vi "Test Query Auth.vi"() -> ()   [LabVIEW 2020]
uses:
  HTTP Server/Trace Log.ctl
  HTTP Server/Trace Item.ctl
  HTTP Server/Processing Step.ctl
  <vilib>/IlluminatedG/IG HTTP Utils/HTTP Utils/Method.ctl
  TestQueryAuth/TestQueryAuth.lvclass
  C:/dev/IlluminatedG/lv-http-server/HTTP Server/Handler/Handler.lvclass
  QueryAuthController/QueryAuthController.lvclass
  HTTP Server/Server/Add Connection Handler.vi
  HTTP Server/Server/Add Request Handler.vi
  HTTP Server/Server/Add Route Handler.vi
  HTTP Server/Server/Add Controller Handler.vi
  HTTP Server/Server/Add Controller.vi
  HTTP Server/Server/Add Response Handler.vi
  HTTP Server/Server/Add Complete Handler.vi
  HTTP Server/Server/Add Exception Handler.vi
  HTTP Server/Connection Handler/Connection Handler.lvclass
  HTTP Server/Request Handler/Request Handler.lvclass
  HTTP Server/Route Handler/Route Handler.lvclass
  HTTP Server/Controller Handler/Controller Handler.lvclass
  HTTP Server/Controller/Controller.lvclass
  HTTP Server/Response Handler/Response Handler.lvclass
  HTTP Server/Complete Handler/Complete Handler.lvclass
  HTTP Server/Exception Handler/Exception Handler.lvclass
  HTTP Server/Server/Server.lvclass
  HTTP Server/Handler/Handler.lvclass
  HTTP Server/RequestTraceLog/RequestTraceLog.lvclass
  HTTP Server/HTTP Server.lvlib
  <vilib>/IlluminatedG/IG HTTP Utils/HTTP Utils/HTTP Utils.lvlib
panel:
  in  "Refresh Traces":bool
  out "Traces":T1[](array[typedef]) {"Sending" format="%_6f"; "Expires" format="%<%X %x>T"; "Created" format="%<%X %x>T"; "Waiting" format="%_6f"; "Parsing" format="%_6f"; "Processing" format="%_6f"; "Items"."Time" format="%.6f"; "Items"."Duration" format="%.6f"}
  out "error out":errorcluster
  in  "Port":u16=36987
  # "Request"
  # "Response"
  # "Session"
  # "Auth"
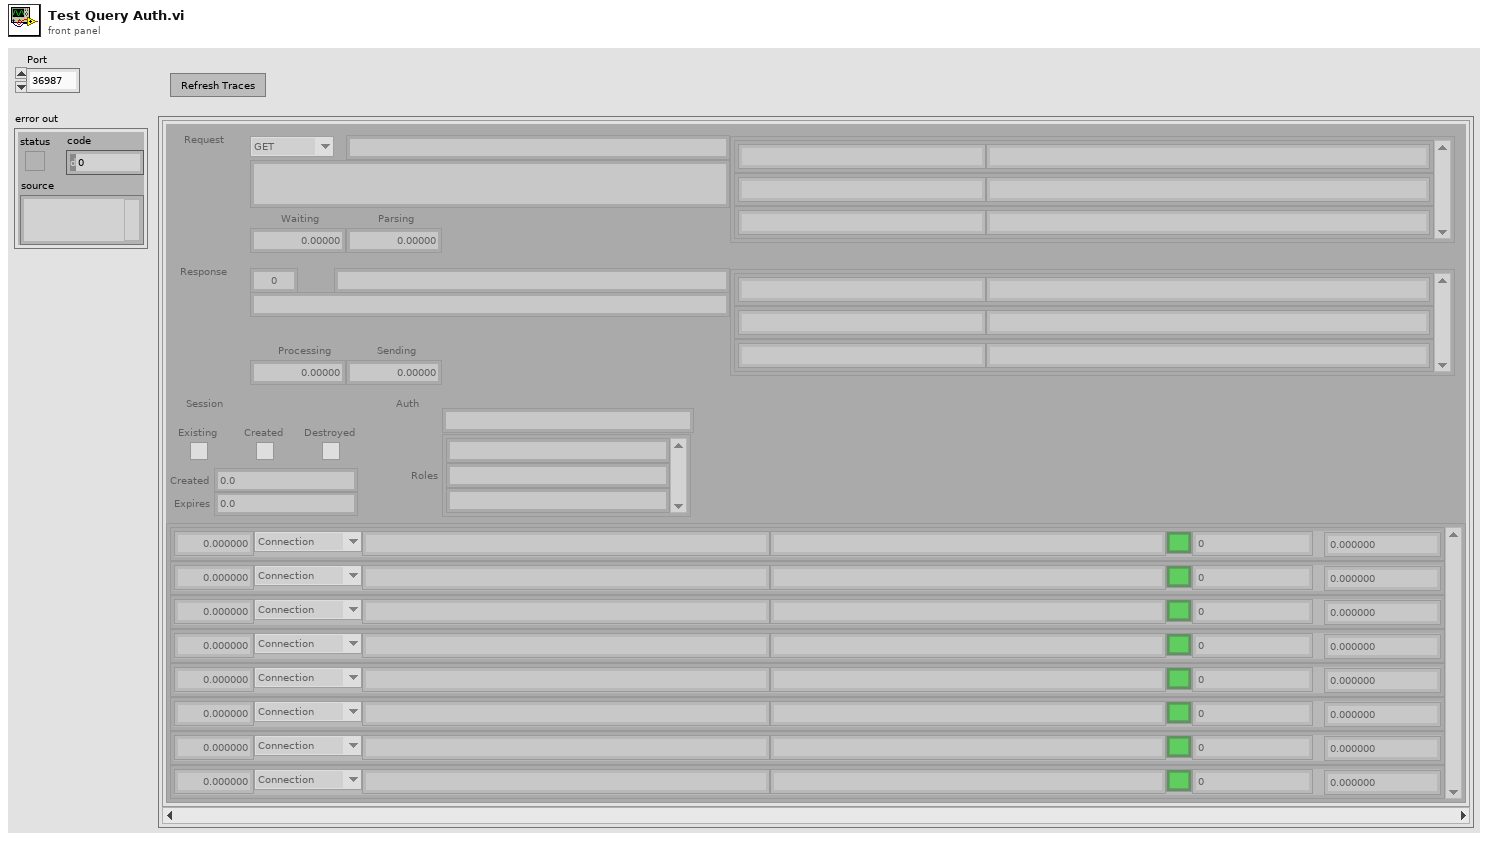
[diagram p1: front panel]
types:
  T1 = typedef "HTTP Server.lvlib/Trace Log.ctl" = cluster{"Items":T2[], "Client":string, "Target":string, "Response Type":string, "Processing":dbl, "Status":u16, "Method":T4, "Content Type":string, "Request Headers":cluster{"Name":string, "Value":string}[], "Parsing":dbl, "Waiting":dbl, "Identity":string, "Existing":bool, "Created":bool, "Destroyed":bool, "Response Headers":cluster{"Name":string, "Value":string}[], "Created":dbl, "Expires":dbl, "Roles":string[], "Sending":dbl}
  T2 = typedef "HTTP Server.lvlib/Trace Item.ctl" = cluster{"Duration":dbl, "Step":T3, "Class":string, "Info":string, "Status":bool, "Code":i32, "Time":dbl}
  T3 = typedef "HTTP Server.lvlib/Processing Step.ctl" = enum16{"Connection", "Request", "Routing", "Controller Init", "Controller", "Response", "Complete", "Exception"}
  T4 = typedef "HTTP Utils.lvlib/Method.ctl" = enum16{"GET", "HEAD", "POST", "PUT", "DELETE", "CONNECT", "OPTIONS", "TRACE", "PATCH"}
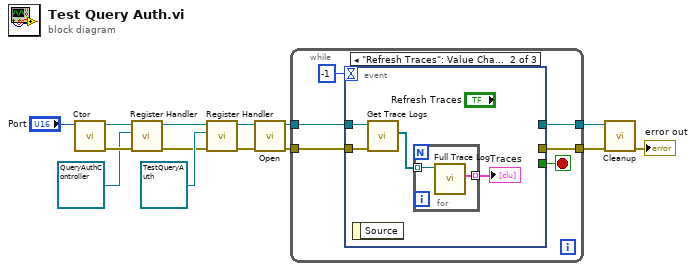
[diagram p0: block diagram]
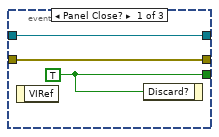
[diagram p2: hidden frame]
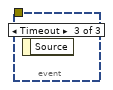
[diagram p3: hidden frame]
diagram:
  n1 = call "Ctor.vi"("Port (8080)"="Port") -> ("error out"=w7:errorcluster, "Server out"=w8:refnum<class "Server.lvclass">)  [unwired: 9 in]
  n2 = call "Register Handler.vi"("error in (no error)"=w7, "Handler"=refnum<class "QueryAuthController.lvclass"> refnum ("QueryAuthController.lvclass"), "Server in"=w8) -> ("error out"=w3:errorcluster, "Server out"=w4:refnum<class "Server.lvclass">)  [unwired: 7 in]
  n3 = call "Register Handler.vi"("error in (no error)"=w3, "Handler"=refnum<class "TestQueryAuth.lvclass"> refnum ("TestQueryAuth.lvclass"), "Server in"=w4) -> ("error out"=w2:errorcluster, "Server out"=w1:refnum<class "Server.lvclass">)  [unwired: 7 in]
  n4 = call "Open.vi"("error in (no error)"=w2, "Server in"=w1) -> ("error out"=w12:errorcluster, "Server out"=w13:refnum<class "Server.lvclass">)  [unwired: 8 in]
  n5 = while {
    tunnel: w13 -> [w18]
    tunnel: w12 -> [w19]
    tunnel: [w17] -> w11
    tunnel: [w16] -> w10
    stop <- w20 stop-if-true
    n6 = event shown="[1] \"Refresh Traces\": Value Change" {
      selector: _ -> [_ _ _]
      dyn-events: _ -> [_ _ _]
      timeout: -1 -> [_ _ _]
      tunnel: [w23 _ _] -> w20
      tunnel: w19 -> [w21 w26 _]
      tunnel: w18 -> [w22 w27 _]
      tunnel: [w22 _ _] -> w17
      tunnel: [w21 _ _] -> w16
      event Panel Close? {
        w23 = TRUE ("Discard?")
        n7 = event-data() -> ()  [unwired: 1 in, 1 out]
        n8 = event-data("Discard?"=w23) -> ()  [unwired: 1 in, 1 out]
      }
      event "Refresh Traces": Value Change {
        n9 = event-data() -> ()  [unwired: 1 in, 1 out]
        n10 = call "Get Trace Logs.vi"("error in (no error)"=w26, "Server in"=w27) -> ("Trace Logs"=w25:refnum<class "RequestTraceLog.lvclass">[])  [unwired: 7 in, 2 out]
        n11 = for {
          tunnel: w25 -> [w29] mode=indexing
          tunnel: [w28] -> w24 mode=indexing
          n12 = call "Full Trace Log.vi"("RequestTraceLog in"=w29) -> ("Trace Log"=w28:T1)  [unwired: 8 in, 2 out]
        }
        "Traces" <- w24
      }
      event Timeout {
        n13 = event-data() -> ()  [unwired: 1 in, 1 out]
      }
    }
  }
  n14 = call "Cleanup.vi"("error in (no error)"=w10, "Server in"=w11) -> ("error out"=→"error out":errorcluster)  [unwired: 9 in]
